vi "cal_para_to_string_pos.vi"(0 "Bool Disable Command":string="OFF", 1 "Enum":T1, 5 "1st sub node x position":i32, 7 "Last Control Position":cluster{"Left":i32, "Top":i32}, 9 "Last Function  Position":cluster{"Left":i32, "Top":i32}, 11 "error in":errorcluster) -> (6 "Bool Node BD Position/Enable String Position":cluster{"1st sub node x position":i32, i32}, 8 "Control BD Position":cluster{"1st sub node x position":i32, i32}, 10 "BD Constant Position/Disable String Position":cluster{"1st sub node x position":i32, i32}, 15 "error out":errorcluster)   [LabVIEW 2018]
uses:
  TypeDefinitions/sub_position_type.ctl
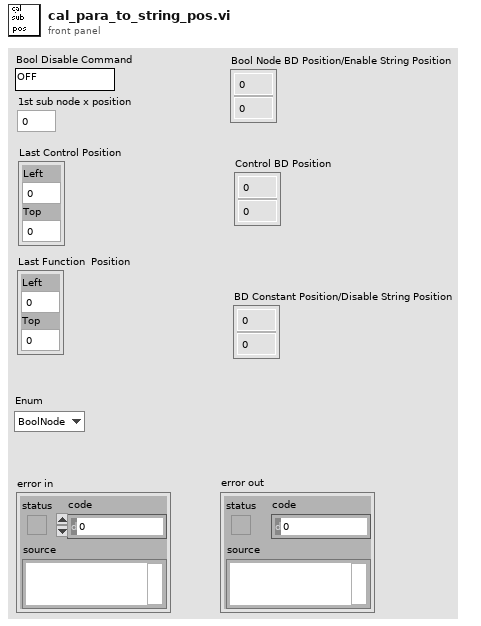
[diagram p1: front panel]
types:
  T1 = typedef "sub_position_type.ctl" = enum16{"BoolNode", "BoolConst", "RingConstNode", "Numeri/String"}
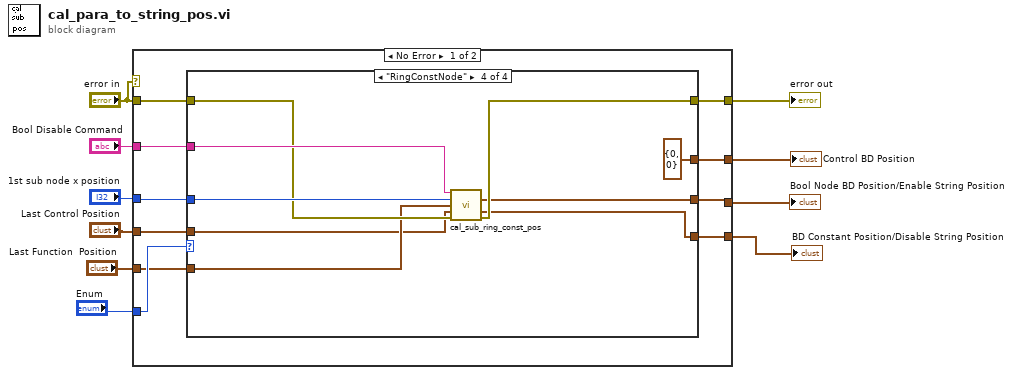
[diagram p0: block diagram]
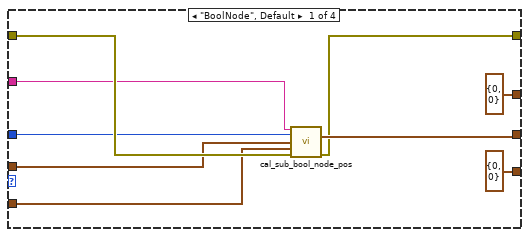
[diagram p2: hidden frame]
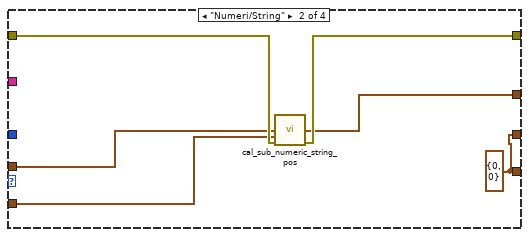
[diagram p3: hidden frame]
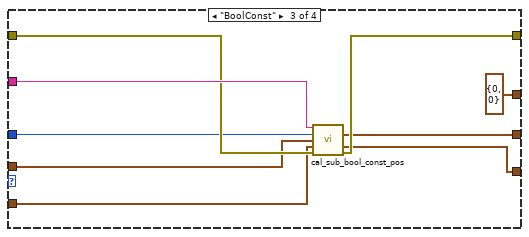
[diagram p4: hidden frame]
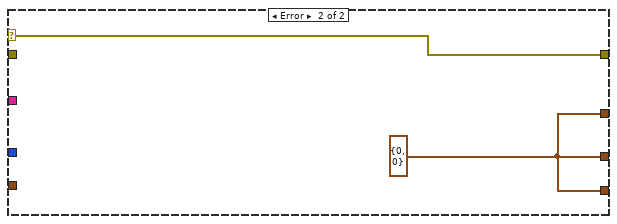
[diagram p5: hidden frame]
diagram:
  n1 = case shown="No Error" "error in" {
    selector: "error in" -> [_ w55]
    tunnel: [w17 w55] -> w10
    tunnel: "error in" -> [w18 _]
    tunnel: "Last Function  Position" -> [w12 _]
    tunnel: "Bool Disable Command" -> [w19 _]
    tunnel: "1st sub node x position" -> [w14 _]
    tunnel: [w15 w54] -> w6
    tunnel: "Enum" -> [w20 _]
    tunnel: [w16 w54] -> w3
    tunnel: "Last Control Position" -> [w13 _]
    tunnel: [w11 w54] -> w1
    frame No Error {
      n2 = case shown="\"RingConstNode\"" w20 {
        tunnel: w19 -> [w26 _ w44 w53]
        tunnel: w18 -> [w27 w35 w43 w51]
        tunnel: [w28 w34 w42 w50] -> w17
        tunnel: [cluster{"Left":i32, "Top":i32} {"Left"=0, "Top"=0} ("BD Constant Position") w30 w41 w48] -> w16
        tunnel: [w29 w30 w40 w49] -> w15
        tunnel: w14 -> [w25 _ w39 w52]
        tunnel: w13 -> [w22 w33 w38 w45]
        tunnel: w12 -> [w24 w32 w37 w46]
        tunnel: [cluster{"1st sub node x position":i32, i32} {"1st sub node x position"=0, 0} ("Ccontrol BD Position") w31 cluster{"1st sub node x position":i32, i32} {"1st sub node x position"=0, 0} ("Ccontrol BD Position") cluster{"1st sub node x position":i32, i32} {"1st sub node x position"=0, 0} ("Ccontrol BD Position")] -> w11
        frame "BoolNode", Default {
          n3 = call "cal_sub_bool_node_pos.vi"("Bool Disable Command"=w26, "1st sub node x position"=w25, "Last Control  Position"=w22, "Last Function  Position"=w24, "error in"=w27) -> ("Bool Node BD Position"=w29:cluster{"1st sub node x position":i32, i32}, "error out"=w28:errorcluster)  [unwired: 9 out]
        }
        frame "Numeri/String" {
          w30 = cluster{"Left":i32, "Top":i32} {"Left"=0, "Top"=0} ("BD Constant Position")
          n4 = call "cal_sub_numeric_string_pos.vi"("Last Control  Position"=w33, "Last Function  Position"=w32, "error in"=w35) -> ("Ccontrol BD Position"=w31:cluster{"1st sub node x position":i32, i32}, "error out"=w34:errorcluster)  [unwired: 1 in, 10 out]
        }
        frame "BoolConst" {
          n5 = call "cal_sub_bool_const_pos.vi"("Disable String"=w44, "1st sub node x position"=w39, "Last Control Position"=w38, "Last Function Position"=w37, "error in"=w43) -> ("Enable String Position"=w40:cluster{"Left":i32, "Top":i32}, "Disable String Position"=w41:cluster{"Left":i32, "Top":i32}, "error out"=w42:errorcluster)  [unwired: 8 out]
        }
        frame "RingConstNode" {
          n6 = call "cal_sub_ring_const_pos.vi"("BD Text"=w53, "1st sub node x position"=w52, "Last Function Position"=w46, "Last Control Position"=w45, "error in"=w51) -> ("BD Node Position"=w49:cluster{"1st sub node x position":i32, i32}, "BD Constant Position"=w48:cluster{i32, i32}, "error out"=w50:errorcluster)  [unwired: 8 out]
        }
      }
    }
    frame Error {
      w54 = cluster{"1st sub node x position":i32, i32} {"1st sub node x position"=0, 0}
    }
  }
  "error out" <- w10
  "Bool Node BD Position/Enable String Position" <- w6
  "BD Constant Position/Disable String Position" <- w3
  "Control BD Position" <- w1
